vi "Data Reader.vi"() -> ()   [LabVIEW 2014]
panel:
  in  "Amount of Decimation":dbl
  in  "Sample Rate":dbl
  in  "Amount of Points":dbl
  out "File Path Indicator":path
  in  "File Path Control":path
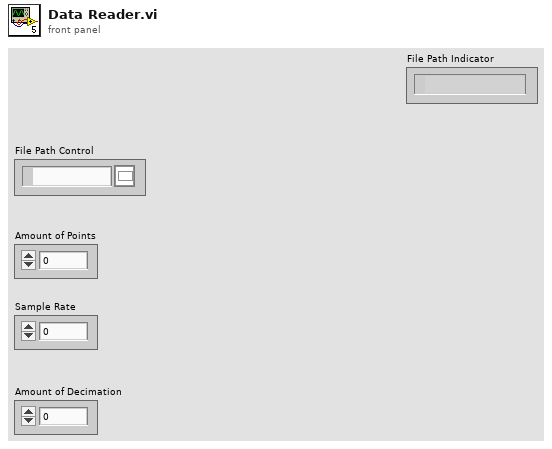
[diagram p1: front panel]
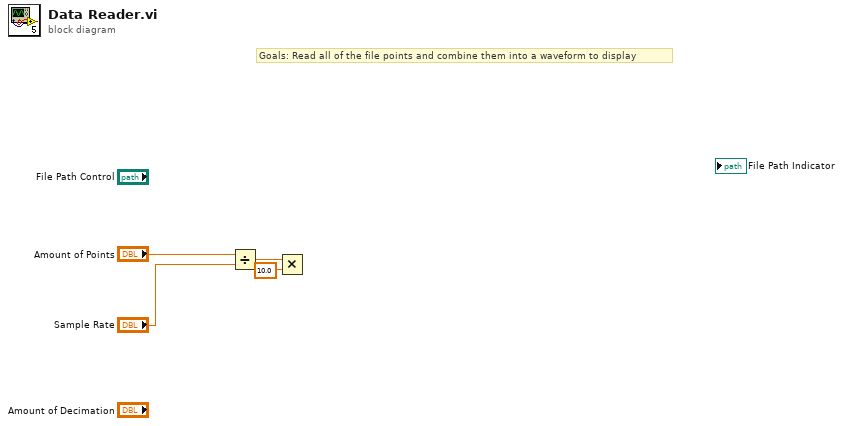
[diagram p0: block diagram]
diagram:
  # "Goals: Read all of the file points and combine them into a waveform to display"
  n1 = Divide(x="Amount of Points", y="Sample Rate") -> (x/y=w2:dbl)
  n2 = Multiply(x=w2, y=10.0) -> ()  [unwired: 1 out]
